vi "MeasuringDevice.GetDepedencies.vi"(8 "error in (no error)":errorcluster, 11 "MeasuringDevice":refnum<class "MeasuringDevice.lvclass">) -> (0 "error out":errorcluster, 2 "Dependencies":T1, 3 "MeasuringDevice":refnum<class "MeasuringDevice.lvclass">)   [LabVIEW 2017, in "MeasuringDevice.lvclass"]
uses:
  MeasuringDevice.lvclass
  Typedefs/Dependencies--Cluster.ctl
  CircularBuffer/CircularBuffer.lvclass
  MeasuringDevice.lvclass/MeasuringDevice.ctl
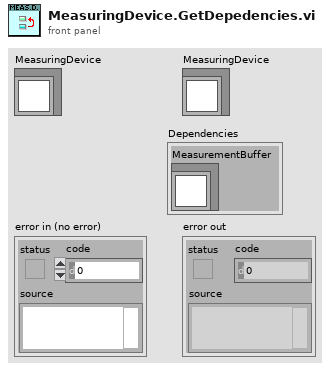
[diagram p1: front panel]
types:
  T1 = typedef "MeasuringDevice.lvclass/Dependencies--Cluster.ctl" = cluster{"MeasurementBuffer":refnum<class "CircularBuffer.lvclass">}
  T2 = typedef "MeasuringDevice.lvclass/PrivateData--Ref.ctl" = refnum<data-value>
  T3 = typedef "MeasuringDevice.lvclass/PrivateData--Cluster.ctl" = cluster{"Public Events":T4, "Private Events":T5, "Dependencies":T1}
  T4 = typedef "MeasuringDevice.lvclass/PublicEvents--Cluster.ctl" = cluster{"MeasurementCompleted":refnum<user-event>}
  T5 = typedef "MeasuringDevice.lvclass/PrivateEvents--Cluster.ctl" = cluster{"MakeMeasurement":refnum<user-event>}
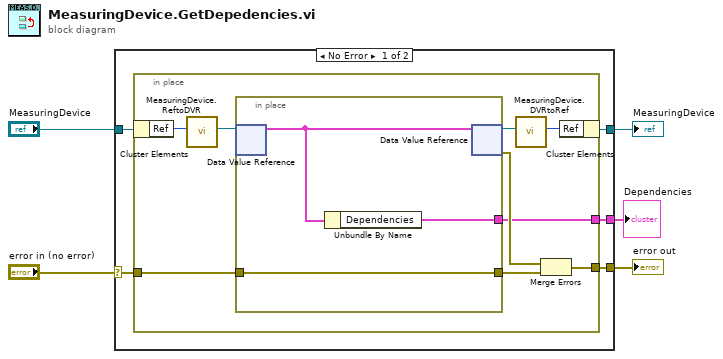
[diagram p0: block diagram]
diagram:
  n1 = case shown="No Error" "error in (no error)" {
    selector: "error in (no error)" -> [w8 w23]
    tunnel: "MeasuringDevice" -> [w10 w24]
    tunnel: [w9 w24] -> w3
    tunnel: [w7 w23] -> w2
    tunnel: [w6 _] -> w1
    frame No Error {
      n2 = in-place {
        in-place-border: w8 -> [w15]
        in-place-border: [w12] -> w7
        in-place-border: [w11] -> w6
        n3 = in-place-cluster #1(w10) -> ("Ref"=w19:u32)
        n4 = call "MeasuringDevice.ReftoDVR.vi"("Ref"=w19) -> ("Ref"=w17:T2)  [unwired: 10 in]
        n5 = in-place {
          in-place-border: w15 -> [w22]
          in-place-border: [w22] -> w14
          in-place-border: [w21] -> w11
          n6 = in-place-dvr #2(w17) -> (w20:T3)  [unwired: 1 out]
          n7 = Unbundle By Name(w20) -> ("Dependencies"=w21:T1)
          n8 = in-place-dvr #2(w20) -> (w16:T2, w13:errorcluster)
        }
        n9 = call "MeasuringDevice.DVRtoRef.vi"("Ref"=w16) -> ("Ref"=w18:u32)  [unwired: 10 in]
        n10 = Merge Errors(w13, w14) -> (w12:errorcluster)
        n11 = in-place-cluster #1("Ref"=w18) -> (w9:refnum<class "MeasuringDevice.lvclass">)
      }
    }
    frame Error {
    }
  }
  "error out" <- w2
  "MeasuringDevice" <- w3
  "Dependencies" <- w1
